vi "AlliGator Phasor Plot Display Mouse Down-Up Event Monitoring.vi"(0 "Phasor Plot Display Event Registration":refnum<event-registration>, 5 "Phasor Plot Display Refnum":T1, 11 "Error In":errorcluster, 12 "Look for Mouse Down(T)/Up(F)":bool) -> (4 "Phasor Plot Display Event Registration":refnum<event-registration>, 15 "Error Out":errorcluster)   [LabVIEW 2021, in "AlliGator Phasor Plot.lvlib"]
doc: "Handles event registration for mouse moves in the Phasor Plot image."
uses:
  Image/Image Control Refnum.ctl
  AlliGator Phasor Plot.lvlib
  Image/Image.lvlib
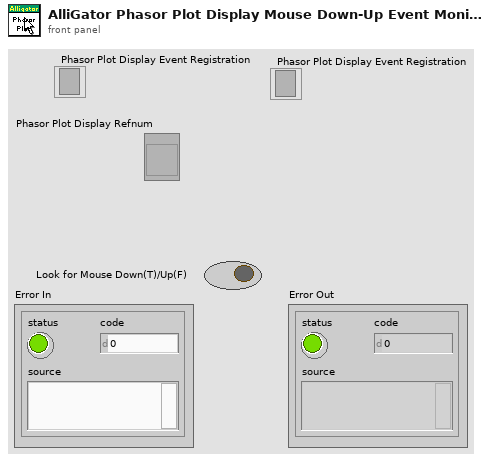
[diagram p1: front panel]
types:
  T1 = typedef "Image.lvlib/Image Control Refnum.ctl" = refnum<vi>
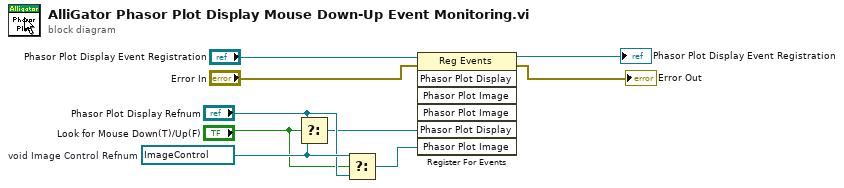
[diagram p0: block diagram]
diagram:
  w9 = refnum<vi> refnum  # void Image Control Refnum
  n1 = Select(t="Phasor Plot Display Refnum", s="Look for Mouse Down(T)/Up(F)", f=w9) -> (s? t:f=w2:T1)
  n2 = Select(t=w9, s="Look for Mouse Down(T)/Up(F)", f="Phasor Plot Display Refnum") -> (s? t:f=w1:T1)
  n3 = register-events(reference="Phasor Plot Display Event Registration", error in="Error In", w2, w1) -> (reference out=→"Phasor Plot Display Event Registration":refnum<event-registration>, error out=→"Error Out":errorcluster)  [unwired: 3 in]
